vi "tcpServerStateMachine.vi"(8 "error in (no error)":errorcluster, 10 "tcpServerQueue":refnum<queue>, 11 "TcpServer in":refnum<class "TcpServer.lvclass">) -> (0 "error out":errorcluster, 3 "TcpServer out":refnum<class "TcpServer.lvclass">)   [LabVIEW 2018, in "TcpServer.lvclass"]
doc: "TCP Server State Machine."
uses:
  TcpServer.lvclass
  TcpServer.lvclass/TcpServer.ctl
  typedef/packetConnIDTypeDef.ctl
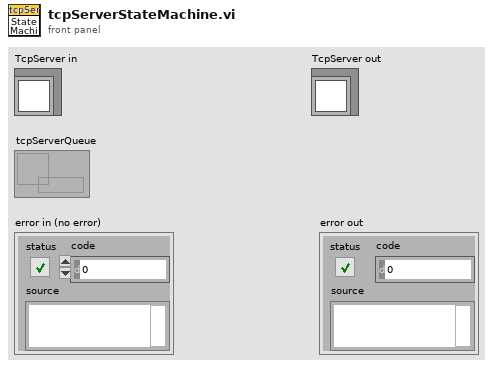
[diagram p1: front panel]
types:
  T1 = enum16{"Standard", "Buffered", "CRLF", "Immediate"}
  T2 = typedef "TcpServer.lvclass/packetConnIDTypeDef.ctl" = cluster{"packet":string, "tcpConnectionID":refnum<k5>, "firstCmdId":bool}
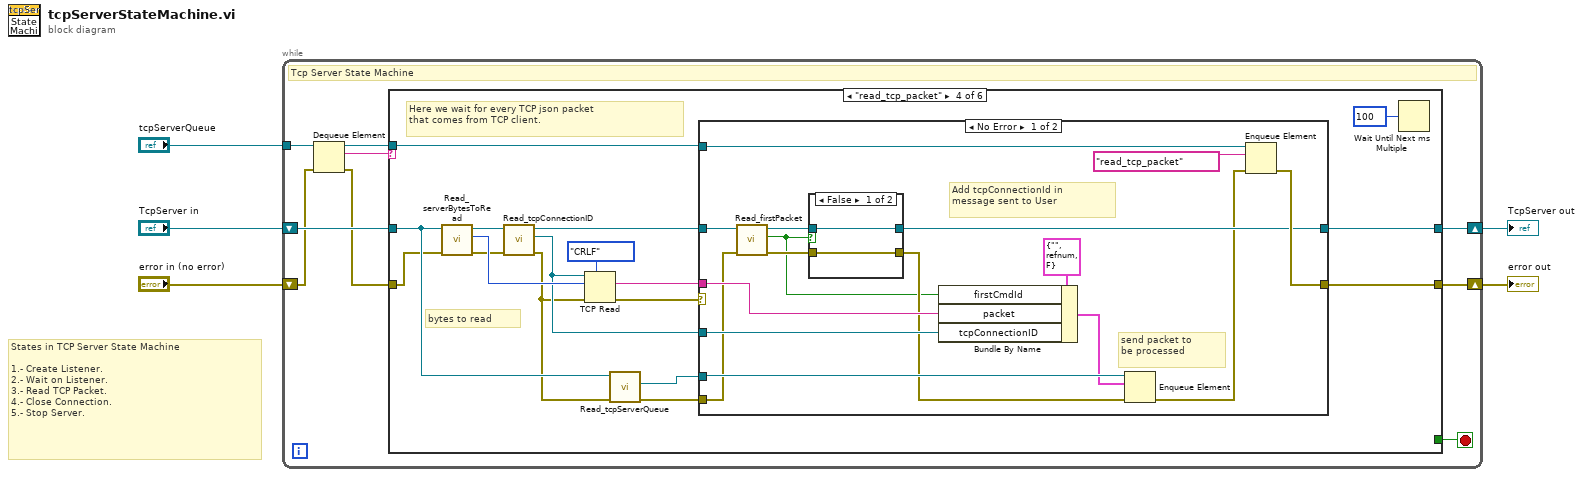
[diagram p0: block diagram]
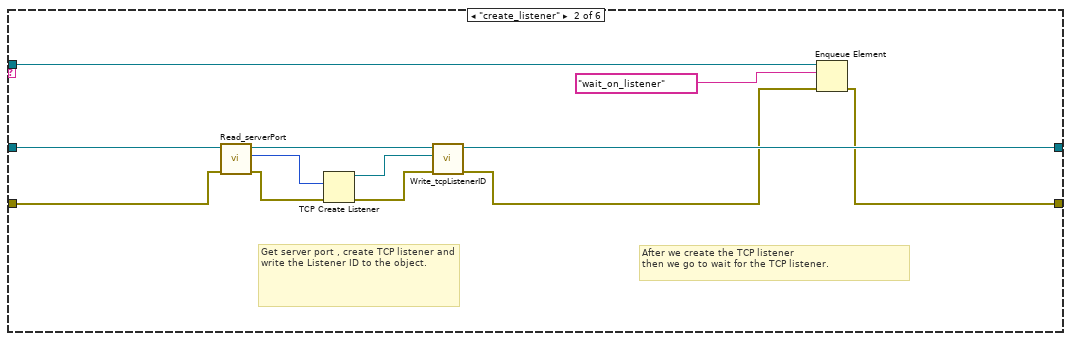
[diagram p3: hidden frame]
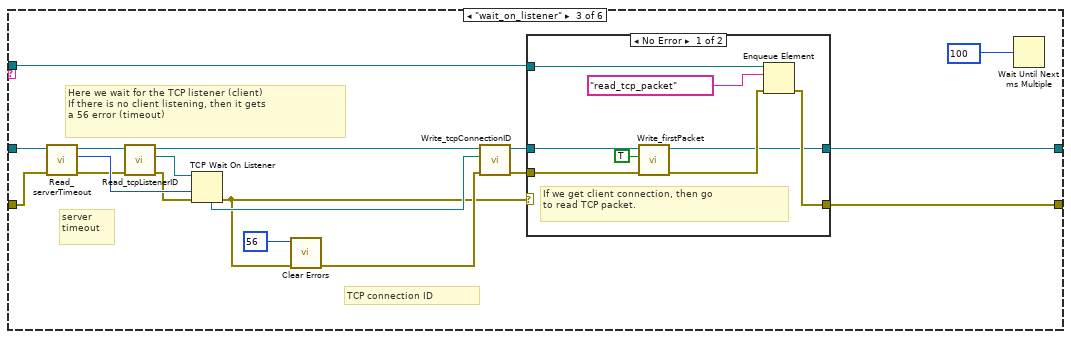
[diagram p4: hidden frame]
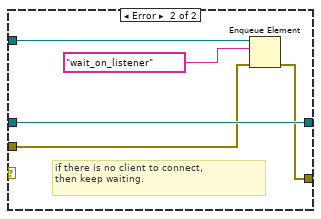
[diagram p5: hidden frame]
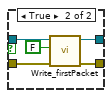
[diagram p6: hidden frame]
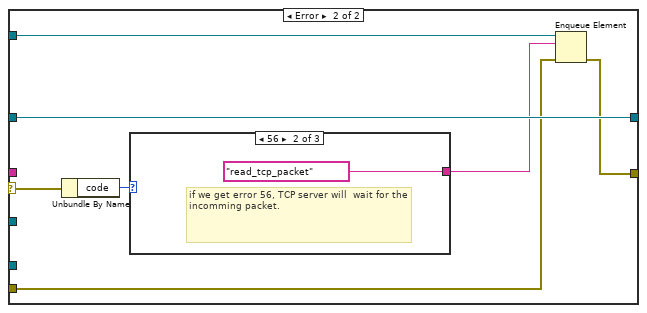
[diagram p7: hidden frame]
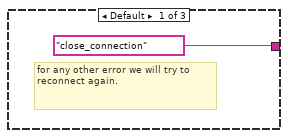
[diagram p8: hidden frame]
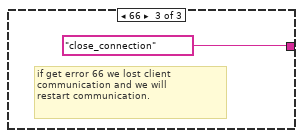
[diagram p9: hidden frame]
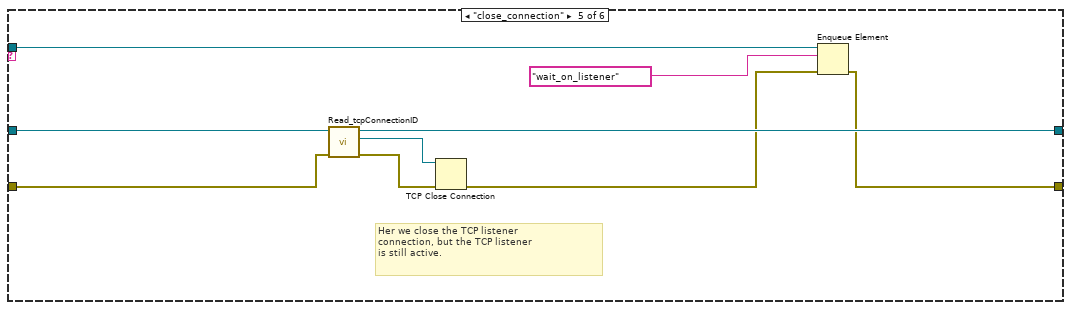
[diagram p10: hidden frame]
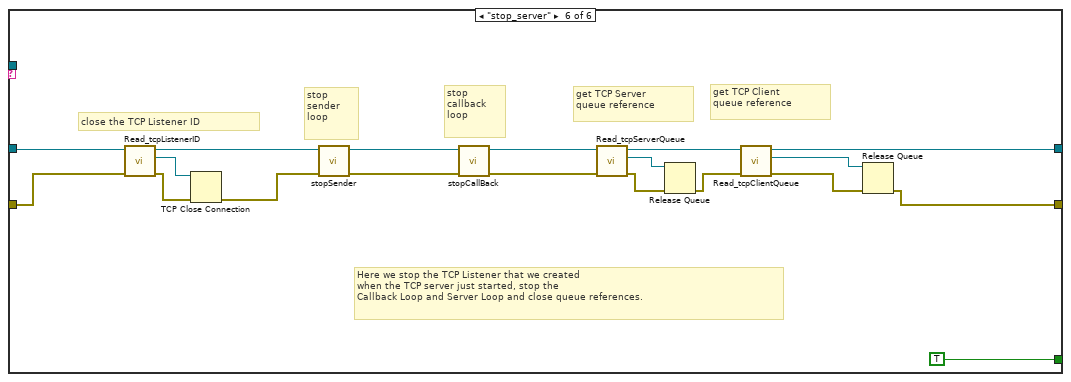
[diagram p11: hidden frame]
diagram:
  # "States in TCP Server State Machine\n\n1.- Create Listener.\n2.- Wait on Listener.\n3.- Read TCP Packet.\n4.- Close Connection.\n5.- Stop Server."
  n1 = while {
    tunnel: "tcpServerQueue" -> [w14]
    shift-right: [w12] -> w1
    shift-left: "TcpServer in" -> [w13]
    shift-right: [w8] -> w4
    shift-left: "error in (no error)" -> [w7]
    stop <- w9 stop-if-true
    # "Tcp Server State Machine"
    n2 = Dequeue Element(queue=w14, error in (no error)=w7) -> (queue out=w11:refnum<queue>, element=w10:string, error out=w6:errorcluster)  [unwired: 1 in, 1 out]
    n3 = case shown="\"read_tcp_packet\"" w10 {
      tunnel: w13 -> [w16 w26 w43 w72 w118 w136]
      tunnel: [w16 w22 w42 w69 w115 w131] -> w12
      tunnel: w11 -> [_ w21 w41 w61 w117 _]
      tunnel: [_ _ _ _ _ TRUE] -> w9
      tunnel: w6 -> [w15 w19 w37 w67 w113 w127]
      tunnel: [w15 w17 w30 w60 w110 w119] -> w8
      frame Default {
        # "Do notihig for now."
      }
      frame "create_listener" {
        # "After we create the TCP listener\nthen we go to wait for the TCP listener."
        # "Get server port , create TCP listener and write the Listener ID to the object."
        n4 = call "Read_serverPort.vi"("error in (no error)"=w19, "tcpServer in"=w26) -> ("error out"=w27:errorcluster, "serverPort"=w28:u16, "tcpServer out"=w25:refnum<class "TcpServer.lvclass">)  [unwired: 7 in]
        n5 = TCP Create Listener(8:w27, 10:w28) -> (0:w23:errorcluster, 3:w24:refnum<k5>)  [unwired: 3 in, 1 out]
        n6 = call "Write_tcpListenerID.vi"("error in (no error)"=w23, "tcpListenerID"=w24, "tcpServer in"=w25) -> ("error out"=w18:errorcluster, "tcpServer out"=w22:refnum<class "TcpServer.lvclass">)  [unwired: 7 in]
        n7 = Enqueue Element(queue=w21, element="wait_on_listener", error in (no error)=w18) -> (error out=w17:errorcluster)  [unwired: 1 in, 2 out]
      }
      frame "wait_on_listener" {
        # "Here we wait for the TCP listener (client)\nIf there is no client listening, then it gets\na 56 error (timeout)"
        # "TCP connection ID"
        # "server\ntimeout"
        n8 = call "Read_serverTimeout.vi"("error in (no error)"=w37, "tcpServer in"=w43) -> ("error out"=w36:errorcluster, "serverTimeout"=w44:i32, "tcpServer out"=w45:refnum<class "TcpServer.lvclass">)  [unwired: 7 in]
        n9 = call "Read_tcpListenerID.vi"("error in (no error)"=w36, "tcpServer in"=w45) -> ("error out"=w35:errorcluster, "tcpListenerID"=w46:refnum<k5>, "tcpServer out"=w40:refnum<class "TcpServer.lvclass">)  [unwired: 7 in]
        n10 = TCP Wait On Listener(8:w35, 9:w44, 11:w46) -> (0:w32:errorcluster, 4:w38:refnum<k5>)  [unwired: 1 in, 3 out]
        n11 = call <vilib>:"Clear Errors.vi"("error in (no error)"=w32, "specific error code to clear (0: all)"=56) -> ("error out"=w33:errorcluster)  [unwired: 4 in, 1 out]
        n12 = call "Write_tcpConnectionID.vi"("error in (no error)"=w33, "tcpConnectionID"=w38, "TcpServer in"=w40) -> ("error out"=w31:errorcluster, "TcpServer out"=w39:refnum<class "TcpServer.lvclass">)  [unwired: 7 in]
        n13 = case shown="No Error" w32 {
          tunnel: w39 -> [w49 w59]
          tunnel: [w48 w59] -> w42
          tunnel: w41 -> [w53 w58]
          tunnel: w31 -> [w52 w56]
          tunnel: [w51 w55] -> w30
          frame No Error {
            # "If we get client connection, then go \nto read TCP packet."
            n14 = call "Write_firstPacket.vi"("error in (no error)"=w52, "firstPacket"=TRUE, "TcpServer in"=w49) -> ("error out"=w50:errorcluster, "TcpServer out"=w48:refnum<class "TcpServer.lvclass">)  [unwired: 7 in]
            n15 = Enqueue Element(queue=w53, element="read_tcp_packet", error in (no error)=w50) -> (error out=w51:errorcluster)  [unwired: 1 in, 2 out]
          }
          frame Error {
            # "if there is no client to connect, \nthen keep waiting."
            n16 = Enqueue Element(queue=w58, element="wait_on_listener", error in (no error)=w56) -> (error out=w55:errorcluster)  [unwired: 1 in, 2 out]
          }
        }
        n17 = Wait Until Next ms Multiple(millisecond multiple=u32 100) -> ()  [unwired: 1 out]
      }
      frame "read_tcp_packet" {
        # "Here we wait for every TCP json packet\nthat comes from TCP client."
        # "bytes to read"
        n18 = call "Read_serverBytesToRead.vi"("error in (no error)"=w67, "tcpServer in"=w72) -> ("error out"=w68:errorcluster, "serverBytesToRead"=w73:i32, "tcpServer out"=w71:refnum<class "TcpServer.lvclass">)  [unwired: 7 in]
        n19 = call "Read_tcpConnectionID.vi"("error in (no error)"=w68, "TcpServer in"=w71) -> ("error out"=w63:errorcluster, "tcpConnectionID"=w64:refnum<k5>, "TcpServer out"=w70:refnum<class "TcpServer.lvclass">)  [unwired: 7 in]
        n20 = TCP Read(connection ID=w64, bytes to read=w73, error in (no error)=w63, 7:T1."CRLF" ("mode (standard)")) -> (data out=w76:string, error out=w74:errorcluster)  [unwired: 1 in, 1 out]
        n21 = call "Read_tcpServerQueue.vi"("error in (no error)"=w63, "tcpServer in"=w72) -> ("error out"=w62:errorcluster, "tcpServerQueue"=w66:refnum<queue>)  [unwired: 7 in, 1 out]
        n22 = case shown="No Error" w74 {
          selector: w74 -> [_ w106]
          tunnel: w76 -> [w89 _]
          tunnel: w66 -> [w92 _]
          tunnel: w70 -> [w91 w104]
          tunnel: [w81 w104] -> w69
          tunnel: w64 -> [w88 _]
          tunnel: w62 -> [w82 w101]
          tunnel: w61 -> [w86 w103]
          tunnel: [w84 w100] -> w60
          frame No Error {
            # "Add tcpConnectionId in\nmessage sent to User"
            # "send packet to\nbe processed"
            n23 = call "Read_firstPacket.vi"("error in (no error)"=w82, "TcpServer in"=w91) -> ("error out"=w79:errorcluster, "firstPacket"=w77:bool, "TcpServer out"=w83:refnum<class "TcpServer.lvclass">)  [unwired: 7 in]
            n24 = case shown="False" w77 {
              tunnel: w83 -> [w94 w99]
              tunnel: [w94 w98] -> w81
              tunnel: w79 -> [w93 w96]
              tunnel: [w93 w95] -> w78
              frame False {
              }
              frame True {
                n25 = call "Write_firstPacket.vi"("error in (no error)"=w96, "firstPacket"=FALSE, "TcpServer in"=w99) -> ("error out"=w95:errorcluster, "TcpServer out"=w98:refnum<class "TcpServer.lvclass">)  [unwired: 7 in]
              }
            }
            n26 = Bundle By Name(cluster=T2 {"packet"="", "tcpConnectionID"=refnum, "firstCmdId"=FALSE}, "firstCmdId"=w77, "packet"=w89, "tcpConnectionID"=w88) -> (w87:T2)
            n27 = Enqueue Element(queue=w92, element=w87, error in (no error)=w78) -> (error out=w80:errorcluster)  [unwired: 1 in, 2 out]
            n28 = Enqueue Element(queue=w86, element="read_tcp_packet", error in (no error)=w80) -> (error out=w84:errorcluster)  [unwired: 1 in, 2 out]
          }
          frame Error {
            n29 = Unbundle By Name(w106) -> ("code"=w105:i32)
            n30 = case shown="56" w105 {
              tunnel: ["close_connection" "read_tcp_packet" "close_connection"] -> w102
              frame Default {
                # "for any other error we will try to reconnect again."
              }
              frame 56 {
                # "if we get error 56, TCP server will  wait for the incomming packet."
              }
              frame 66 {
                # "if get error 66 we lost client \ncommunication and we will\nrestart communication."
              }
            }
            n31 = Enqueue Element(queue=w103, element=w102, error in (no error)=w101) -> (error out=w100:errorcluster)  [unwired: 1 in, 2 out]
          }
        }
        n32 = Wait Until Next ms Multiple(millisecond multiple=u32 100) -> ()  [unwired: 1 out]
      }
      frame "close_connection" {
        # "Her we close the TCP listener\nconnection, but the TCP listener\nis still active."
        n33 = call "Read_tcpConnectionID.vi"("error in (no error)"=w113, "TcpServer in"=w118) -> ("error out"=w112:errorcluster, "tcpConnectionID"=w114:refnum<k5>, "TcpServer out"=w115:refnum<class "TcpServer.lvclass">)  [unwired: 7 in]
        n34 = TCP Close Connection(connection ID=w114, error in (no error)=w112) -> (error out=w111:errorcluster)  [unwired: 1 in, 1 out]
        n35 = Enqueue Element(queue=w117, element="wait_on_listener", error in (no error)=w111) -> (error out=w110:errorcluster)  [unwired: 1 in, 2 out]
      }
      frame "stop_server" {
        # "Here we stop the TCP Listener that we created\nwhen the TCP server just started, stop the \nCallback Loop and Server Loop and close queue references."
        # "close the TCP Listener ID"
        # "stop\nsender\nloop"
        # "stop\ncallback\nloop"
        # "get TCP Client \nqueue reference"
        # "get TCP Server \nqueue reference"
        n36 = call "Read_tcpListenerID.vi"("error in (no error)"=w127, "tcpServer in"=w136) -> ("error out"=w126:errorcluster, "tcpListenerID"=w137:refnum<k5>, "tcpServer out"=w129:refnum<class "TcpServer.lvclass">)  [unwired: 7 in]
        n37 = TCP Close Connection(connection ID=w137, error in (no error)=w126) -> (error out=w125:errorcluster)  [unwired: 1 in, 1 out]
        n38 = call "stopSender.vi"("error in (no error)"=w125, "TcpServer in"=w129) -> ("error out"=w124:errorcluster, "TcpServer out"=w130:refnum<class "TcpServer.lvclass">)  [unwired: 8 in]
        n39 = call "stopCallBack.vi"("error in (no error)"=w124, "TcpServer in"=w130) -> ("error out"=w123:errorcluster, "TcpServer out"=w128:refnum<class "TcpServer.lvclass">)  [unwired: 8 in]
        n40 = call "Read_tcpServerQueue.vi"("error in (no error)"=w123, "tcpServer in"=w128) -> ("error out"=w122:errorcluster, "tcpServerQueue"=w134:refnum<queue>, "tcpServer out"=w133:refnum<class "TcpServer.lvclass">)  [unwired: 7 in]
        n41 = Release Queue(queue=w134, error in (no error)=w122) -> (error out=w121:errorcluster)  [unwired: 1 in, 2 out]
        n42 = call "Read_tcpClientQueue.vi"("error in (no error)"=w121, "tcpServer in"=w133) -> ("error out"=w120:errorcluster, "tcpClientQueue"=w132:refnum<queue>, "tcpServer out"=w131:refnum<class "TcpServer.lvclass">)  [unwired: 7 in]
        n43 = Release Queue(queue=w132, error in (no error)=w120) -> (error out=w119:errorcluster)  [unwired: 1 in, 2 out]
      }
    }
  }
  "error out" <- w4
  "TcpServer out" <- w1
